vi "Poincare_spheric_to_cartesian.vi"(3 "phi":dbl, 4 "theta (xy-ebene)":dbl, 5 "Magnitude (mT)":dbl) -> (0 "Z":dbl, 1 "Y":dbl, 2 "X":dbl)   [LabVIEW 2024]
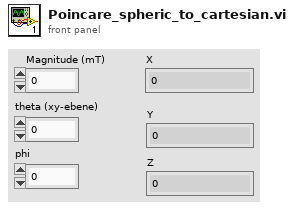
[diagram p1: front panel]
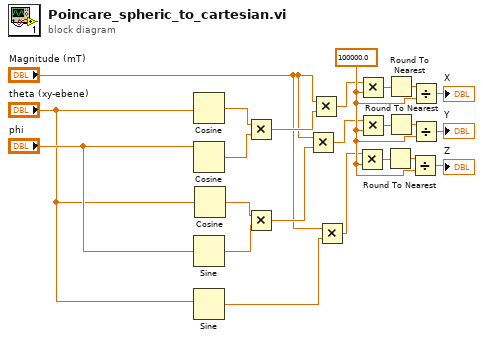
[diagram p0: block diagram]
diagram:
  w14 = 100000.0 ("y")
  n1 = Cosine(x="theta (xy-ebene)") -> (cos(x)=w13:dbl)
  n2 = Cosine(x="phi") -> (cos(x)=w12:dbl)
  n3 = Sine(x="phi") -> (sin(x)=w8:dbl)
  n4 = Sine(x="theta (xy-ebene)") -> (sin(x)=w3:dbl)
  n5 = Cosine(x="theta (xy-ebene)") -> (cos(x)=w9:dbl)
  n6 = Multiply(x=w13, y=w12) -> (x*y=w11:dbl)
  n7 = Multiply(x=w9, y=w8) -> (x*y=w7:dbl)
  n8 = Multiply(x="Magnitude (mT)", y=w7) -> (x*y=w5:dbl)
  n9 = Multiply(x="Magnitude (mT)", y=w11) -> (x*y=w10:dbl)
  n10 = Multiply(x="Magnitude (mT)", y=w3) -> (x*y=w1:dbl)
  n11 = Multiply(x=w1, y=w14) -> (x*y=w17:dbl)
  n12 = Multiply(x=w10, y=w14) -> (x*y=w23:dbl)
  n13 = Multiply(x=w5, y=w14) -> (x*y=w19:dbl)
  n14 = Round To Nearest(number=w17) -> (nearest integer value=w16:dbl)
  n15 = Round To Nearest(number=w23) -> (nearest integer value=w22:dbl)
  n16 = Round To Nearest(number=w19) -> (nearest integer value=w20:dbl)
  n17 = Divide(x=w16, y=w14) -> (x/y=→"Z":dbl)
  n18 = Divide(x=w22, y=w14) -> (x/y=→"X":dbl)
  n19 = Divide(x=w20, y=w14) -> (x/y=→"Y":dbl)
